vi "DB Tools Format Datetime String (Seconds).vi"(1 "seconds (now)":u32) -> (0 "date/time string":string)   [LabVIEW 2012, in "NI_Database_API_64.lvlib"]
doc: "Returns a string containing the formatted date and time, and identifies the string as a date/time string so other VIs can interpret this string. Wire data to the input of this VI to determine the polymorphic instance to use or manually select the instance."
uses:
  NI_Database_API_64.lvlib
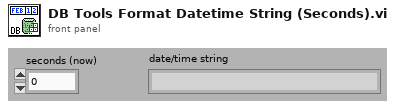
[diagram p1: front panel]
types:
  T1 = typedef "LVDateTimeRec.ctl" = cluster{"fractional second":dbl, "second":i32, "minute":i32, "hour":i32, "day of month":i32, "month":i32, "year":i32, "day of week":i32, "day of year":i32, "DST":i32}
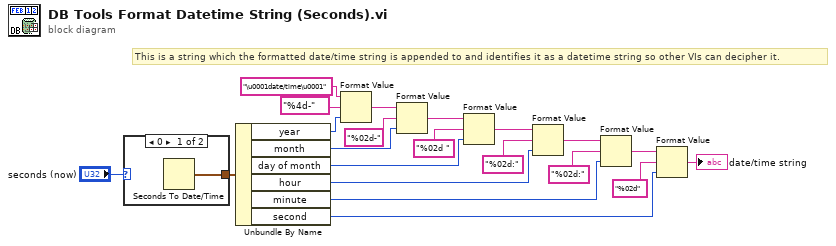
[diagram p0: block diagram]
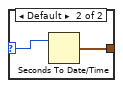
[diagram p2: hidden frame]
diagram:
  # "This is a string which the formatted date/time string is appended to and identifies it as a datetime string so other VIs can decipher it."
  n1 = case shown="0" "seconds (now)" {
    selector: "seconds (now)" -> [_ w24]
    tunnel: [w22 w23] -> w6
    frame 0 {
      n2 = Seconds To Date/Time() -> (date time rec=w22:T1)  [unwired: 2 in]
    }
    frame Default {
      n3 = Seconds To Date/Time(time stamp (now)=w24) -> (date time rec=w23:T1)  [unwired: 1 in]
    }
  }
  n4 = Unbundle By Name(w6) -> ("year"=w9:i32, "month"=w8:i32, "day of month"=w7:i32, "hour"=w21:i32, "minute"=w18:i32, "second"=w17:i32)
  n5 = Format Value(string ("")="\u0001date/time\u0001", format string="%4d-", value (0)=w9) -> (output string=w12:string)
  n6 = Format Value(string ("")=w12, format string="%02d-", value (0)=w8) -> (output string=w11:string)
  n7 = Format Value(string ("")=w11, format string="%02d ", value (0)=w7) -> (output string=w10:string)
  n8 = Format Value(string ("")=w10, format string="%02d:", value (0)=w21) -> (output string=w20:string)
  n9 = Format Value(string ("")=w20, format string="%02d:", value (0)=w18) -> (output string=w19:string)
  n10 = Format Value(string ("")=w19, format string="%02d", value (0)=w17) -> (output string=→"date/time string":string)
